vi "feedforward.vi"() -> ()   [LabVIEW 2015]
uses:
  <vilib>/imath/engines/lvmath2/RunTimeEngine/BuiltInFunctions/is_empty/NIMS_is_empty(GM).vi
  <instcachedir>/0/NIMS_is_empty(GM)_AF8F13F4B7FD436CB1855477E2504B8A.lvgen/NIMS_is_empty(GM)_AF8F13F4B7FD436CB1855477E2504B8A_004.vi
  <vilib>/imath/engines/lvmath2/RunTimeEngine/BuiltInFunctions/rand/NIMS_rand(I32,I32).vi
  <vilib>/imath/engines/lvmath2/RunTimeEngine/ErrorHandling/NIMS_Error From Error Code.vi
  <vilib>/imath/engines/lvmath2/RunTimeEngine/ArithmeticOperatorToken/NIMS_ArithmeticOperator_multmx(M,CV).vi
  <instcachedir>/0/NIMS_ArithmeticOperator_multmx(M,CV)_C9EF95620DE142FBA54888430A25DC18.lvgen/NIMS_ArithmeticOperator_multmx(M,CV)_C9EF95620DE142FBA54888430A25DC18_002.vi
  <vilib>/imathl/engines/lvmath/Functions/Error Handling/Create Error.vi
  <vilib>/imath/engines/lvmath2/RunTimeEngine/ArithmeticOperatorToken/NIMS_ArithmeticOperator_multmx.vi
  <instcachedir>/0/NIMS_ArithmeticOperator_multmx_E413577642394AA3A74EB19F669417B0.lvgen/NIMS_ArithmeticOperator_multmx_E413577642394AA3A74EB19F669417B0_004.vi
  <vilib>/imath/engines/lvmath2/RunTimeEngine/NodeEndStatement/NIMS_NodeEndStatement_Output.vi
  <instcachedir>/0/NIMS_NodeEndStatement_Output_53EC0D466D134D7ABD903AC30B43404B.lvgen/NIMS_NodeEndStatement_Output_53EC0D466D134D7ABD903AC30B43404B_002.vi
  <vilib>/imath/engines/lvmath2/RunTimeEngine/ErrorHandling/NIMS_Finalize Error.vi
panel:
  out "W1":dbl[][](array[numeric])
  out "W2":dbl[][](array[numeric])
  out "Input":dbl[](array[numeric])
  out "Output":dbl[][](array[numeric])
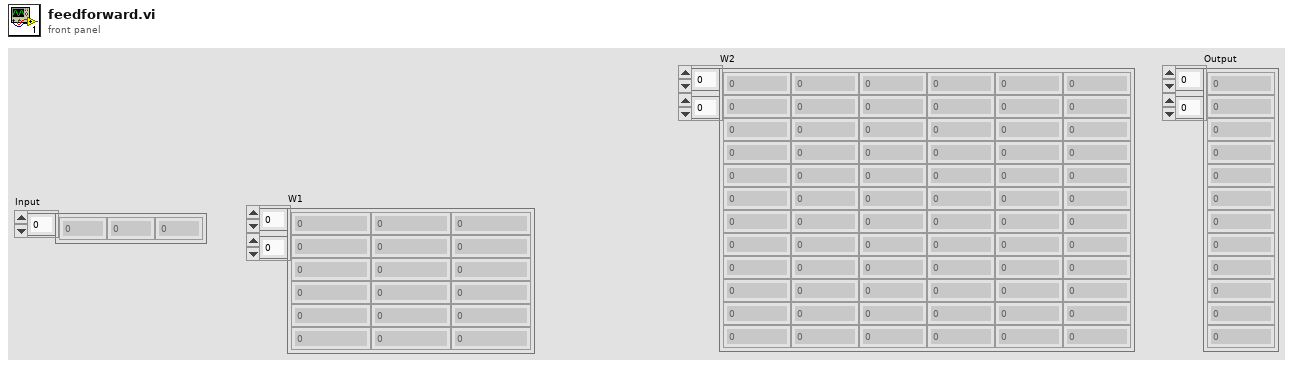
[diagram p1: front panel]
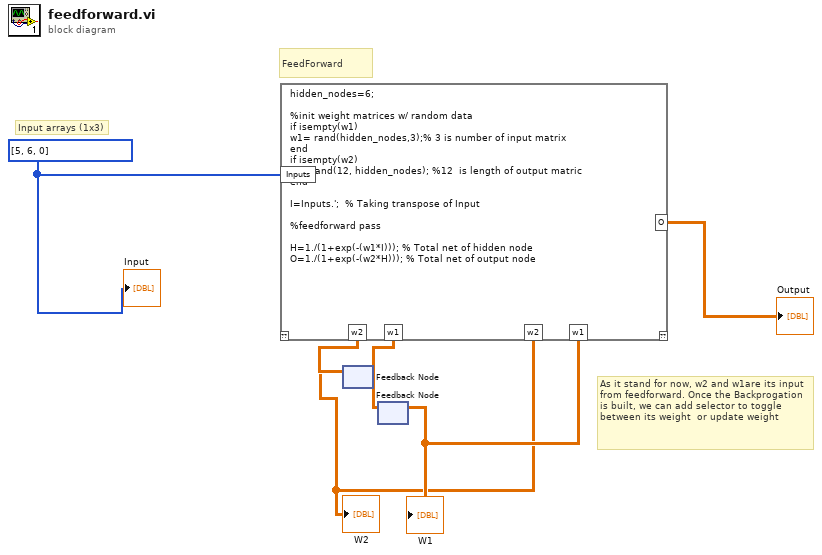
[diagram p0: block diagram]
diagram:
  w6 = i32[] [5, 6, 0]
  # "As it stand for now, w2 and w1are its input from feedforward. Once the Backprogation is built, we can add selector to toggle between its weight  or update weight"
  # "Input arrays (1x3)"
  # "FeedForward"
  n1 = feedback #1() -> (w1:dbl[][])  [unwired: 1 in]
  "W2" <- w1
  n2 = feedback #2() -> (w3:dbl[][])  [unwired: 1 in]
  "W1" <- w3
  n3 = mathscript code="hidden_nodes=6;\n\n%init weight matrices w/ random data\nif isempty(w1)\nw1= rand(hidden_nodes,3);% 3 is number of input matrix\nend\nif isempty(w2)\nw2=rand(12, hidden_nodes); %12  is length of output matric\nend\n\nI=Inputs.';  % Taking transpose of Input\n\n%feedforward pass\n\nH=1./(1+exp(-(w1*I))); % Total net of hidden node \nO=1./(1+exp(-(w2*H))); % Total net of output node"("Inputs"=w6, "w2"=w1, "w1"=w3) -> ("O"=→"Output":dbl[][], "w1"=w4:dbl[][], "w2"=w2:dbl[][])  [unwired: 1 in, 1 out]
  n4 = feedback-in #1(w2) -> ()
  n5 = feedback-in #2(w4) -> ()
  "Input" <- w6
